vi "FrictionCompensatedU.vi"(2 "u_Right":dbl, 3 "Right Lin Vel":dbl, 4 "u_Left":dbl, 5 "Left Lin Vel":dbl) -> (0 "RightU":dbl, 1 "LeftU":dbl)   [LabVIEW 2017]
uses:
  <vilib>/Simulation/Implementation/Shared/SIMSCR Execution Mode.ctl
  <vilib>/Simulation/Scripting/Companion Diagram/SimConfigNode/SimParams.ctl
  <vilib>/Simulation/Scripting/Companion Diagram/SimConfigNode/_simSolvers.ctl
  <vilib>/Simulation/Param Hierarchy/Typedefs/SIMPH Param Control Actions.ctl
  <vilib>/Simulation/Implementation/Shared/NILVSim_ParamChanged.vi
  <vilib>/Simulation/Implementation/Shared/NILVSIM_BeginStep.vi
  <vilib>/Simulation/Implementation/Shared/SIM Is Init or Final Stage.vi
  <vilib>/Simulation/Implementation/Shared/NILVSim_Manager.vi
  <vilib>/Utility/error.llb/Clear Errors.vi
  <vilib>/Simulation/Implementation/Shared/NILVSim_FinalizeModel.vi
  <vilib>/Simulation/Implementation/Shared/SIM Unbundle Sim Info.vi
  <vilib>/Simulation/Implementation/Shared/SIMSH Read Queue.vi
  <vilib>/Simulation/Implementation/Shared/NILVSim_Initialize.vi
  <vilib>/Simulation/Utility/Implementation/NILVSim Get Time and IsAcceptedStep.vi
  <vilib>/Simulation/Implementation/Shared/NILVSim_GetModelError.vi
  <vilib>/Simulation/Implementation/Shared/SIM SimErrorHandler.vi
  <vilib>/Simulation/Implementation/Shared/SIM Bundle Sim Info.vi
  <vilib>/Simulation/Scripting/Companion Diagram/SimConfigNode/SimDog.xnode
  <vilib>/Simulation/Implementation/XNodeFramework/SimXNode/SimX.xnode
  <vilib>/Simulation/Implementation/Shared/NI_SIM_Implementation.lvlib
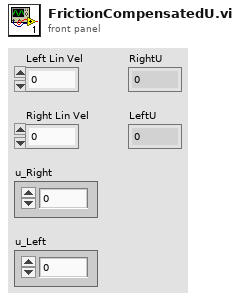
[diagram p1: front panel]
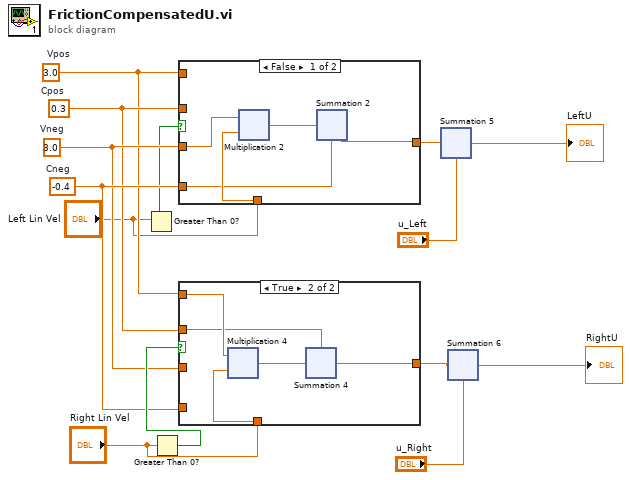
[diagram p0: block diagram]
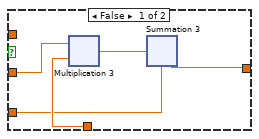
[diagram p2: hidden frame]
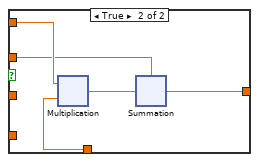
[diagram p3: hidden frame]
diagram:
  w7 = -0.4  # Cneg
  w6 = 3.0  # Vneg
  w5 = 0.3  # Cpos
  w4 = 3.0  # Vpos
  n1 = Greater Than 0?(x="Left Lin Vel") -> (x > 0?=w1:bool)
  n2 = Greater Than 0? ("Greater Than 0? 2")(x="Right Lin Vel") -> (x > 0?=w14:bool)
  n3 = case shown="False" w1 {
    tunnel: w4 -> [_ w30]
    tunnel: w5 -> [_ w27]
    tunnel: w6 -> [w18 _]
    tunnel: w7 -> [w16 _]
    tunnel: "Left Lin Vel" -> [w17 w29]
    tunnel: [w15 w26] -> w8
    frame False {
      n4 = xnode ("Multiplication 2")("Operand1"=w18, "Operand2"=w17) -> ("Result"=w19:dbl)
      n5 = xnode ("Summation 2")("Operand1"=w19, "Operand2"=w16) -> ("Result"=w15:dbl)
    }
    frame True {
      n6 = xnode ("Multiplication")("Operand1"=w30, "Operand2"=w29) -> ("Result"=w28:dbl)
      n7 = xnode ("Summation")("Operand1"=w27, "Operand2"=w28) -> ("Result"=w26:dbl)
    }
  }
  n8 = case "Case Structure 2" shown="True" w14 {
    tunnel: w4 -> [_ w52]
    tunnel: w5 -> [_ w49]
    tunnel: w6 -> [w40 _]
    tunnel: w7 -> [w38 _]
    tunnel: "Right Lin Vel" -> [w39 w51]
    tunnel: [w37 w48] -> w9
    frame False {
      n9 = xnode ("Multiplication 3")("Operand1"=w40, "Operand2"=w39) -> ("Result"=w41:dbl)
      n10 = xnode ("Summation 3")("Operand1"=w41, "Operand2"=w38) -> ("Result"=w37:dbl)
    }
    frame True {
      n11 = xnode ("Multiplication 4")("Operand1"=w52, "Operand2"=w51) -> ("Result"=w50:dbl)
      n12 = xnode ("Summation 4")("Operand1"=w49, "Operand2"=w50) -> ("Result"=w48:dbl)
    }
  }
  n13 = xnode ("Summation 5")("Operand1"=w8, "Operand2"="u_Left") -> ("Result"=→"LeftU":dbl)
  n14 = xnode ("Summation 6")("Operand1"=w9, "Operand2"="u_Right") -> ("Result"=→"RightU":dbl)
